vi "plugins_switch.vi"(6 "error in":errorcluster, 7 "Plugin Pnl":refnum<vi>, 8 "Plugin Index":i32, 9 "Plugins In":T1(array[cluster])) -> (0 "error out":errorcluster, 3 "Plugins Out":T1(array[cluster]))   [LabVIEW 2015]
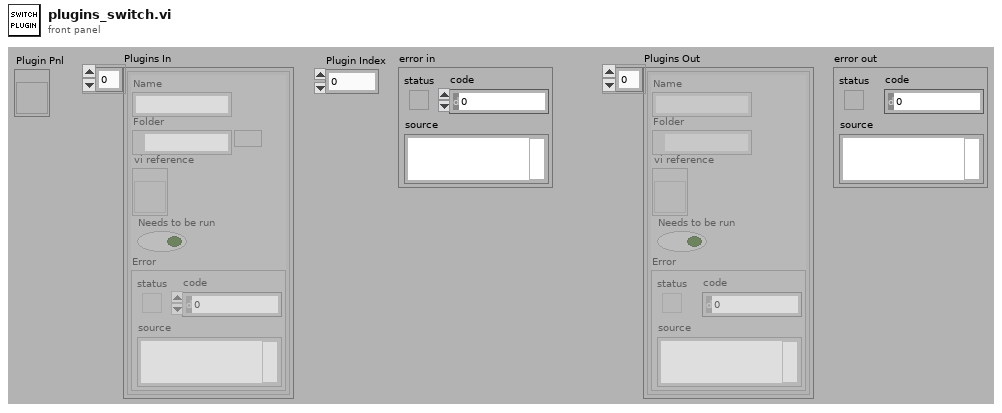
[diagram p1: front panel]
types:
  T1 = cluster{"Name":string, "Folder":path, "vi reference":refnum<vi>, "Needs to be run":bool, "Error":errorcluster}[]
  T2 = cluster{"Name":string, "Folder":path, "vi reference":refnum<vi>, "Needs to be run":bool, "Error":errorcluster}
  T3 = enum32{"Bad", "Idle", "Run top level", "Running"}
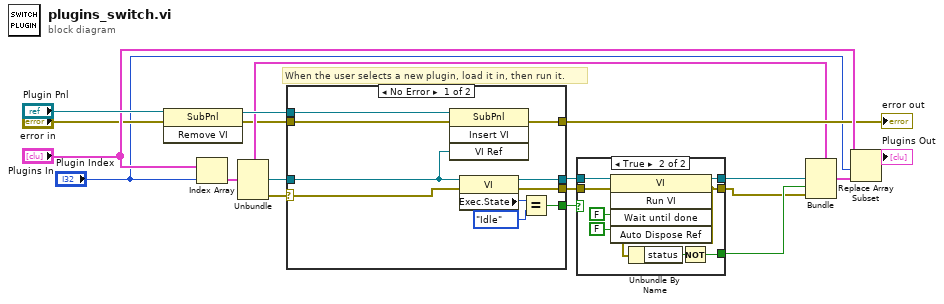
[diagram p0: block diagram]
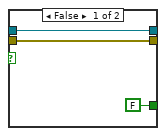
[diagram p2: hidden frame]
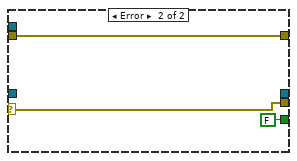
[diagram p3: hidden frame]
diagram:
  # "When the user selects a new plugin, load it in, then run it."
  n1 = invoke on="Invoke Node" class="SubPnl" method="Remove VI"(reference="Plugin Pnl", error in="error in") -> (reference out=w18:refnum<vi>, error out=w6:errorcluster)  [unwired: 1 in, 1 out]
  n2 = Index Array(array="Plugins In", index="Plugin Index") -> (element=w7:T2)
  n3 = Unbundle(w7) -> ("vi reference"=w4:refnum<vi>, "Error"=w5:errorcluster)  [unwired: 3 out]
  n4 = case shown="No Error" w5 {
    selector: w5 -> [w23 w30]
    tunnel: w4 -> [w24 _]
    tunnel: [w26 _] -> w1
    tunnel: [w25 FALSE] -> w3
    tunnel: [w21 w30] -> w2
    tunnel: w6 -> [w22 w29]
    tunnel: [w20 w29] -> w14
    tunnel: w18 -> [w19 _]
    frame No Error {
      n5 = invoke on="Invoke Node" class="SubPnl" method="Insert VI"(reference=w19, error in=w22, "VI Ref"=w24) -> (error out=w20:errorcluster)  [unwired: 1 in, 3 out]
      n6 = property class="VI"(reference=w24, error in=w23) -> (reference out=w26:refnum<vi>, error out=w21:errorcluster, "Exec.State"=w28:T3)
      n7 = Equal?(x=w28, y=T3."Idle" ("Execution:State")) -> (x = y?=w25:bool)
    }
    frame Error {
    }
  }
  "error out" <- w14
  n8 = case shown="True" w3 {
    tunnel: w1 -> [w32 w42]
    tunnel: w2 -> [w34 w41]
    tunnel: [w32 w38] -> w8
    tunnel: [w34 w36] -> w9
    tunnel: [FALSE w35] -> w10
    frame False {
    }
    frame True {
      n9 = invoke class="VI" method="Run VI"(reference=w42, error in=w41, "Wait until done"=FALSE ("Wait Until Done"), "Auto Dispose Ref"=FALSE ("Auto Dispose Reference")) -> (reference out=w38:refnum<vi>, error out=w36:errorcluster)  [unwired: 1 in, 3 out]
      n10 = Unbundle By Name(w36) -> ("status"=w37:bool)
      n11 = Not(x=w37) -> (.not. x?=w35:bool)
    }
  }
  n12 = Bundle(cluster=w7, "vi reference"=w8, "Needs to be run"=w10, "Error"=w9) -> (w11:T2)  [unwired: 2 in]
  n13 = Replace Array Subset(array="Plugins In", new element=w11, index="Plugin Index") -> (→"Plugins Out":T1)
